vi "CR-导丝缺损检测1.vi"(8 "error in (no error)":errorcluster caption="错误输入（无错误）", 11 "名称或相对路径":string="Template Program") -> (0 "error in (no error) 2":errorcluster caption="错误输入（无错误）")   [LabVIEW 2017]
uses:
  Picture/SaveButtom.ctl
  Global System.vi
  <vilib>/Utility/xml.llb/Write to XML File(string).vi
panel:
  in  "获取图像":bool
  in  "ROI获取":bool
  in  "创建模板":bool
  in  "保存图像":bool
  out "添加的路径":path
  in  "刷新":bool
  in  "测试按钮":bool
  in  "保存按钮":bool
  in  "Main":enum32{"主参数", "模板匹配参数 ", "测试效果"}(tab)
  in  "导丝缺损检测1基础参数":T1={"IsNorImage"=TRUE, "Exposure Values"=100289, "ImagePath"=path "C:/Users/hedongpo/Desktop/514-hdp/Alignment Assemble System/Test Picture/B/3.bmp"} caption="参数界面" {"Exposure Values" scale=0.0..200000.0}
  in  "导丝缺损检测1参数":T3={"Rectangle"={"Left"=0, "Top"=0, "Right"=0, "Bottom"=0, "Rotation"=0.0}, "Algorithm "=2, "Parameters"={"Number of Matches Requested"=1, "Minimum Match Score"=800.0, "Angle Ranges"=[{"Start Angle"=-180.0, "End Angle"=180.0}]}, "Advanced Options "=[{"Item"=102, "Value"=10.0}, {"Item"=106, "Value"=300.0}, {"Item"=107, "Value"=0.0}, {"Item"=108, "Value"=6.0}, {"Item"=109, "Value"=1.0}, {"Item"=114, "Value"=25.0}, {"Item"=111, "Value"=20.0}, {"Item"=112, "Value"=10.0}, {"Item"=113, "Value"=20.0}, {"Item"=103, "Value"=1.0}, {"Item"=104, "Value"=20.0}, {"Item"=105, "Value"=0.0}, {"Item"=100, "Value"=5.0}], "模板路径"=path "", "Color Plane "=0} {"Color Plane" items=["Red", "Green", "Blue", "Hue", "Saturation", "Luminance", "Value", "Intensity"]; "Advanced Options"."Item" items=["LD Sampling - Minimum Constrast"=0, "LD Sampling - Enable Subpixel Accuracy"=1, "LD Sampling - Search Strategy"=2, "LD Sampling - Subpixel Iterations"=3, "LD Sampling - Subpixel Tolerance"=4, "LD Sampling - Initial Match List Length"=5, "LD Sampling - Match List Reduction Factor"=6, "LD Sampling - Initial Step Size"=7, "LD Sampling - Intermediate Angular Accuracy"=8, "-"=9, "Pyramid - Max Pyramid Level"=100, "Pyramid - Minimum Contrast"=102, "Pyramid - Enable Subpixel Accuracy"=103, "Pyramid - Subpixel Iterations"=104, "Pyramid - Subpixel Tolerance"=105, "Pyramid - Initial Match List Length"=106, "Pyramid - Match List Reduction Factor"=107, "Pyramid - Intermediate Angular Accuracy"=108, "Pyramid - Process Border Matches"=109, "Pyramid - Min Match Separation Distance"=111, "Pyramid - Min Match Separation Angle"=112, "Pyramid - Max Match Overlap"=113, "Pyramid - Max Cache in MB"=114, "Pyramid - Clear Cache"=115, "-"=116, "Enable Defect Map"=200]; "Algorithm" items=["All", "Low Discrepancy Sampling", "Grayscale Value Pyramid", "Gradients Pyramid"]; "Rectangle"."Rotation" format="%.2f"; "Rectangle"."Left" scale=0.0..1024.0; "Rectangle"."Right" scale=0.0..1024.0}
  out "结果":bool
  out "原始图像":T4(plugin-control)
  out "路径输出":path
  in  "Vision Paramter Save Buttom":T5
  out "system time":string
  in  "取消按钮":bool
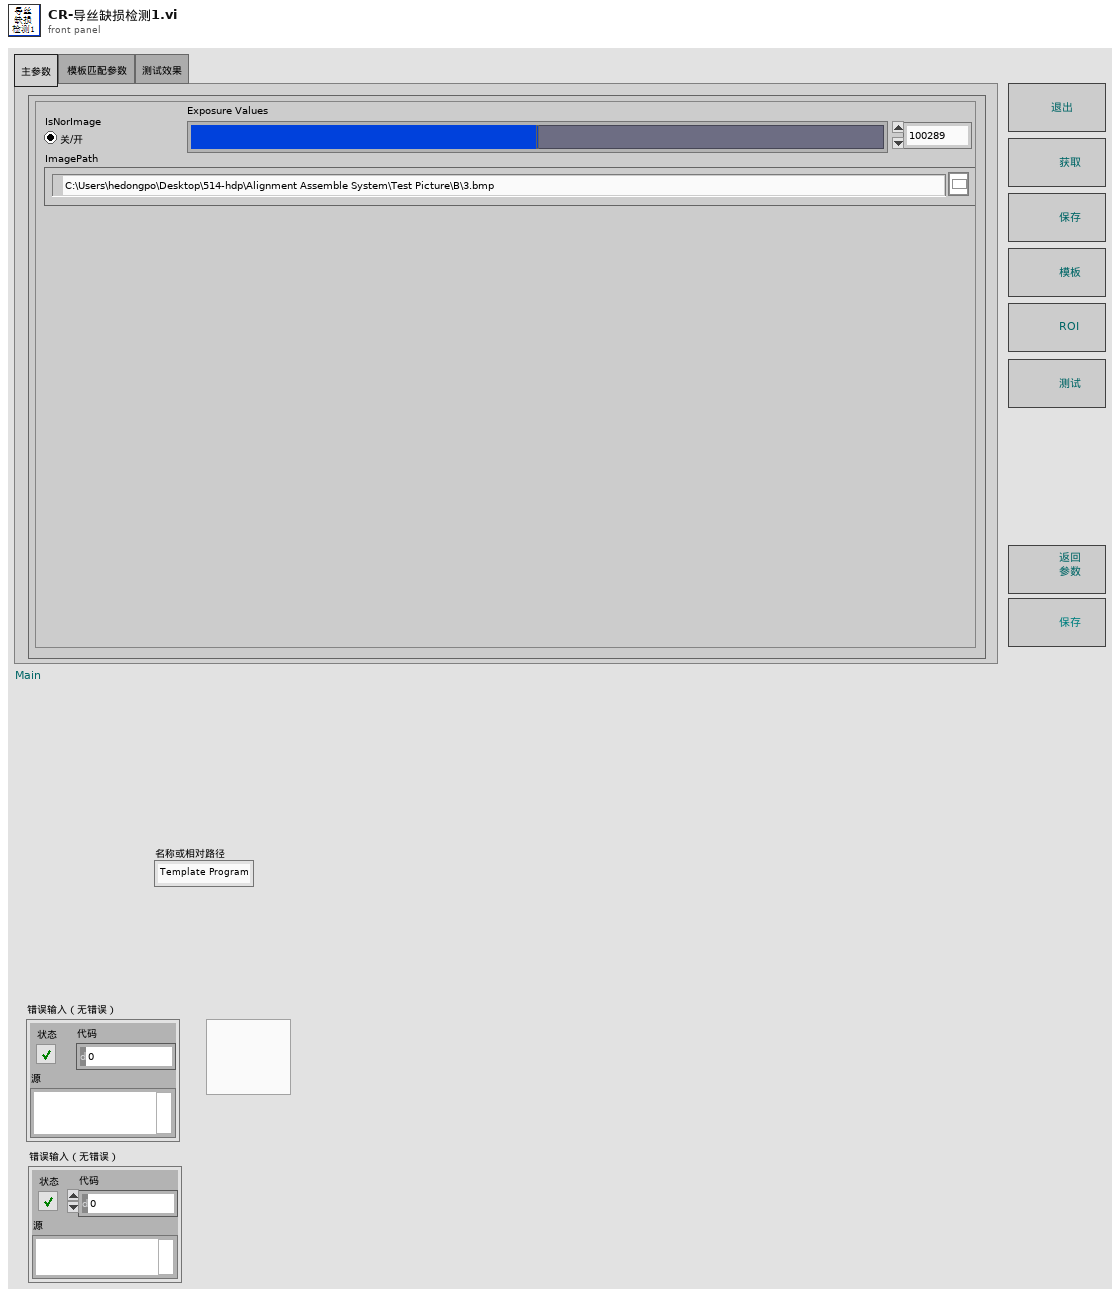
[diagram p1: front panel]
types:
  T1 = cluster{"IsNorImage":bool, "Exposure Values":u32, "ImagePath":path}
  T2 = typedef "IMAQ Rectangle" = cluster{"Left":i32, "Top":i32, "Right":i32, "Bottom":i32, "Rotation":dbl}
  T3 = cluster{"Rectangle":T2, "Algorithm ":i32, "Parameters":cluster{"Number of Matches Requested":i32, "Minimum Match Score":sgl, "Angle Ranges":cluster{"Start Angle":sgl, "End Angle":sgl}[]}, "Advanced Options ":cluster{"Item":u16, "Value":dbl}[], "模板路径":path, "Color Plane ":i32}
  T4 = typedef "IMAQ Image.ctl" = refnum<image>
  T5 = typedef "SaveButtom.ctl" = bool
  T6 = cluster{"index":i32, "this vi":refnum<vi>, "error out":errorcluster}
  T7 = cluster{"master data":string, "priority":u16, "secondary data":string[]}
  T8 = cluster{"case name":string[], "queue array":refnum<queue>[]}
  T9 = cluster{"Global Rectangle":i32[], "Contours":cluster{"Contour Type":u32, "ROI Type":u32, "Points":i32[]}[]}
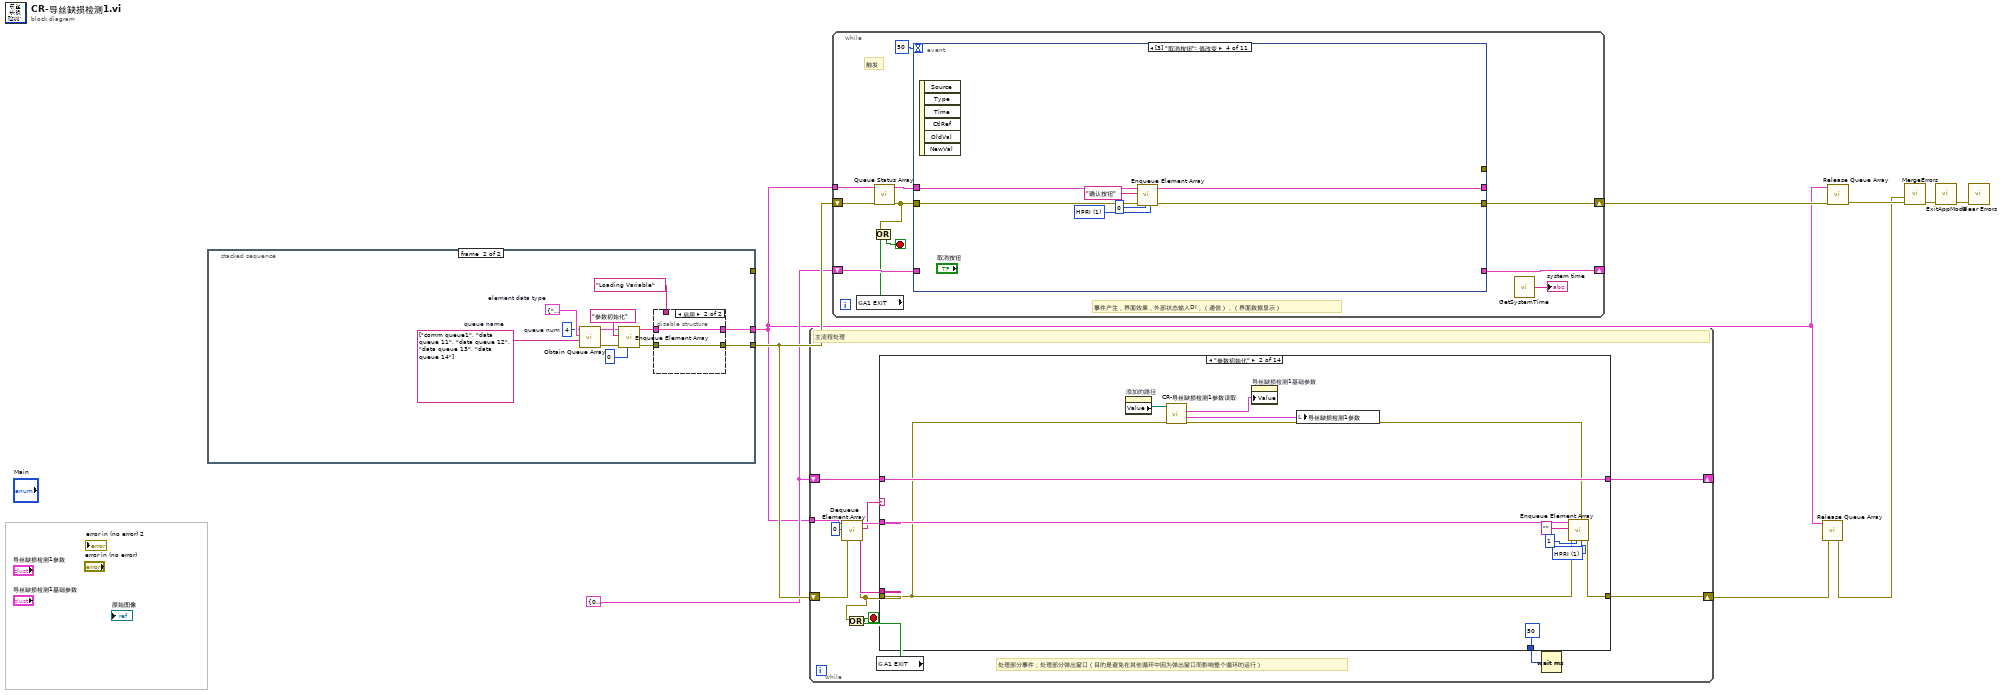
[diagram p0: block diagram]
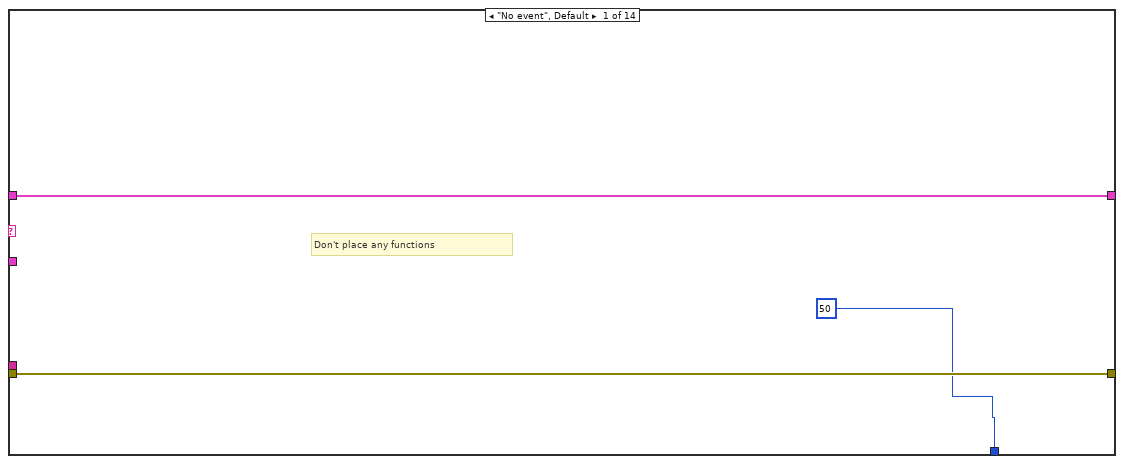
[diagram p2: hidden frame]
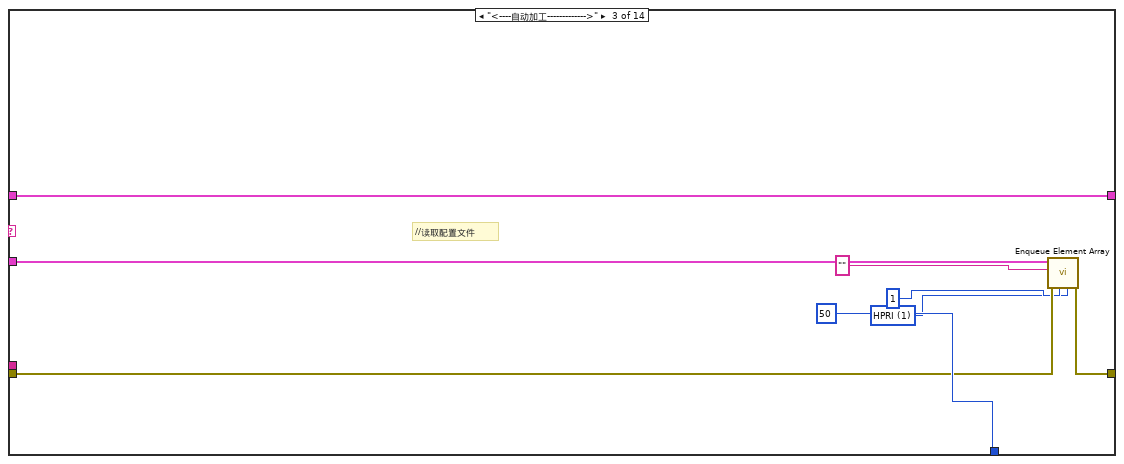
[diagram p3: hidden frame]
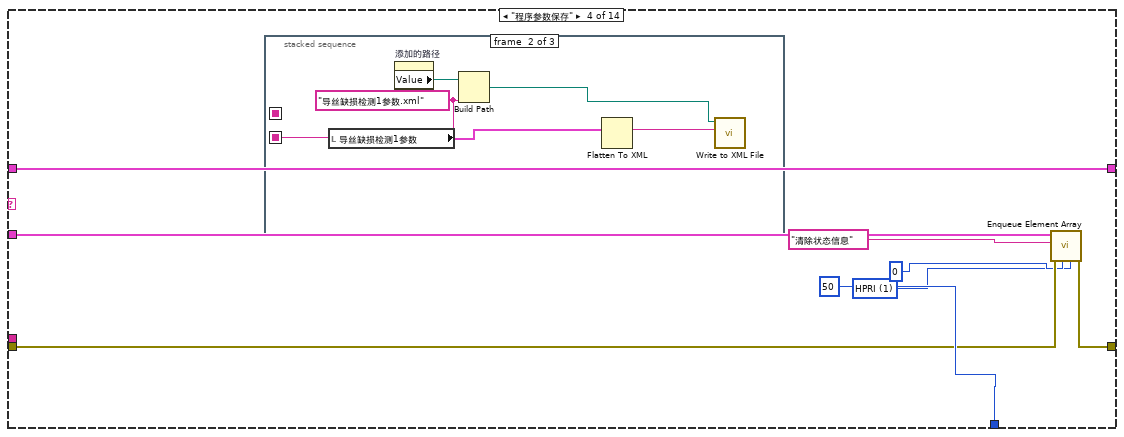
[diagram p4: hidden frame]
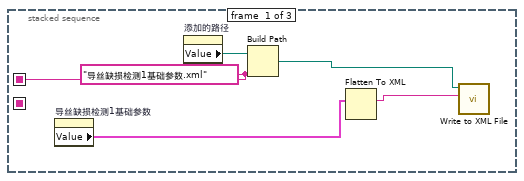
[diagram p5: hidden frame]
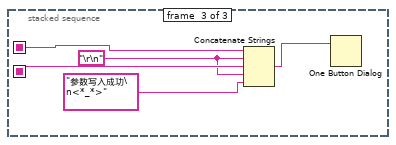
[diagram p6: hidden frame]
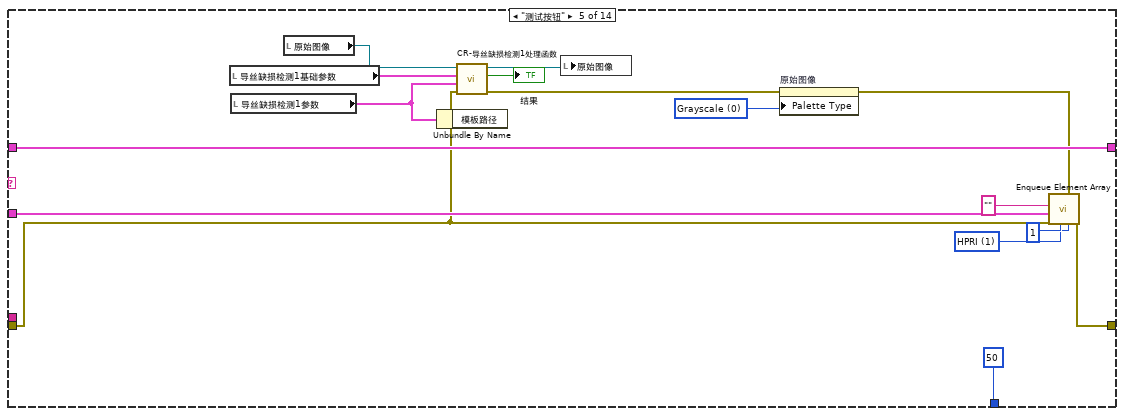
[diagram p7: hidden frame]
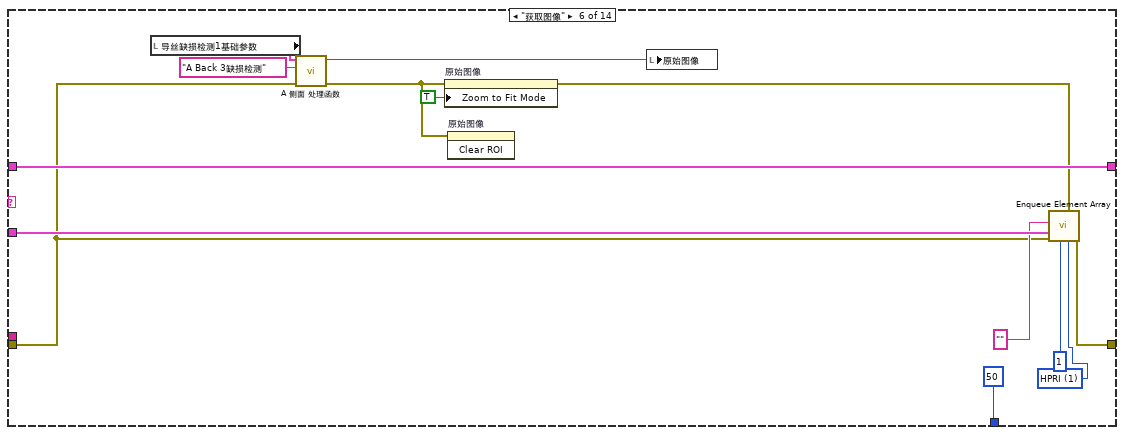
[diagram p8: hidden frame]
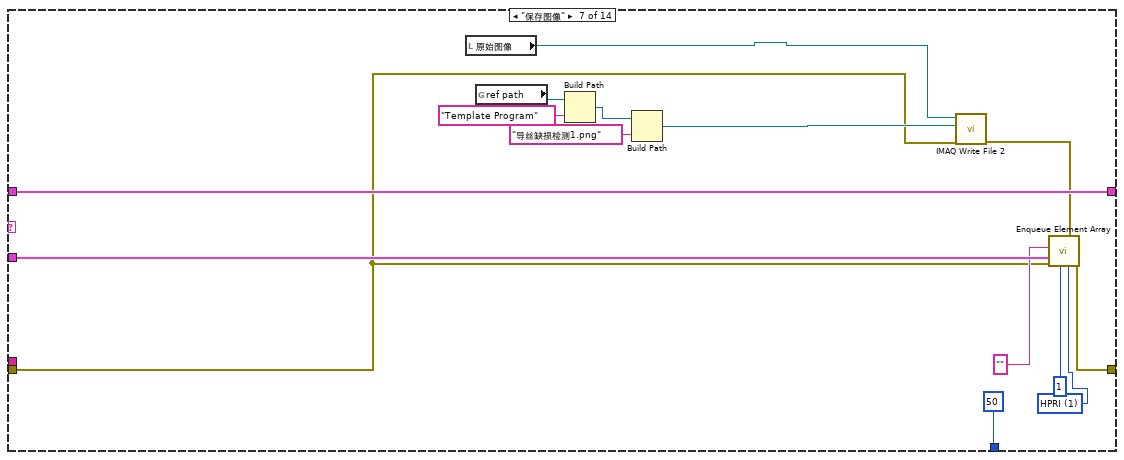
[diagram p9: hidden frame]
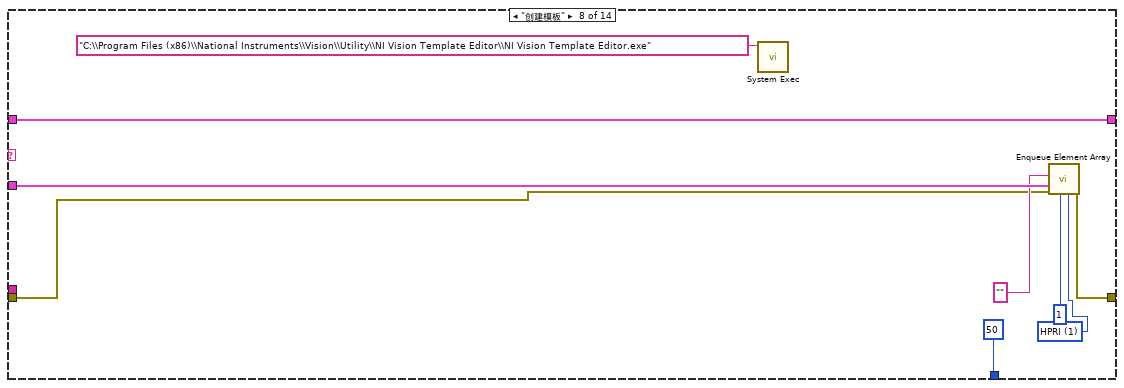
[diagram p10: hidden frame]
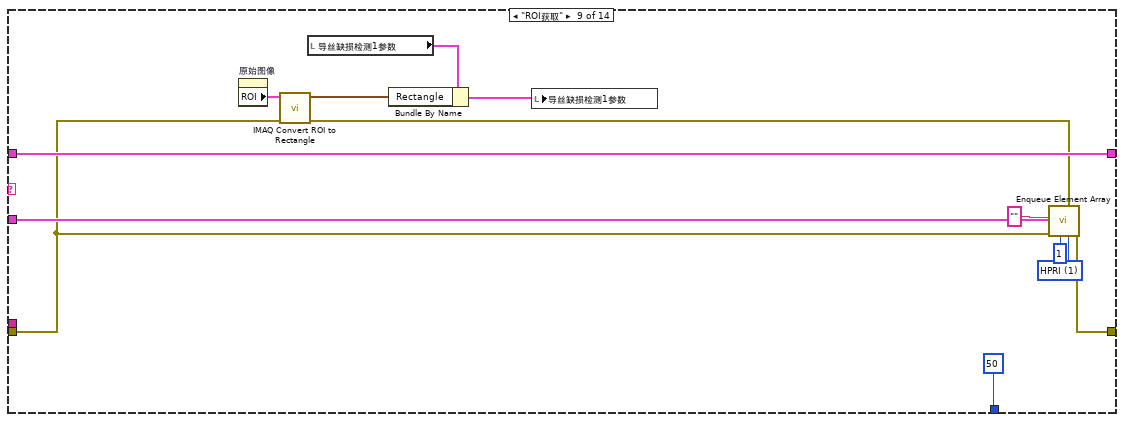
[diagram p11: hidden frame]
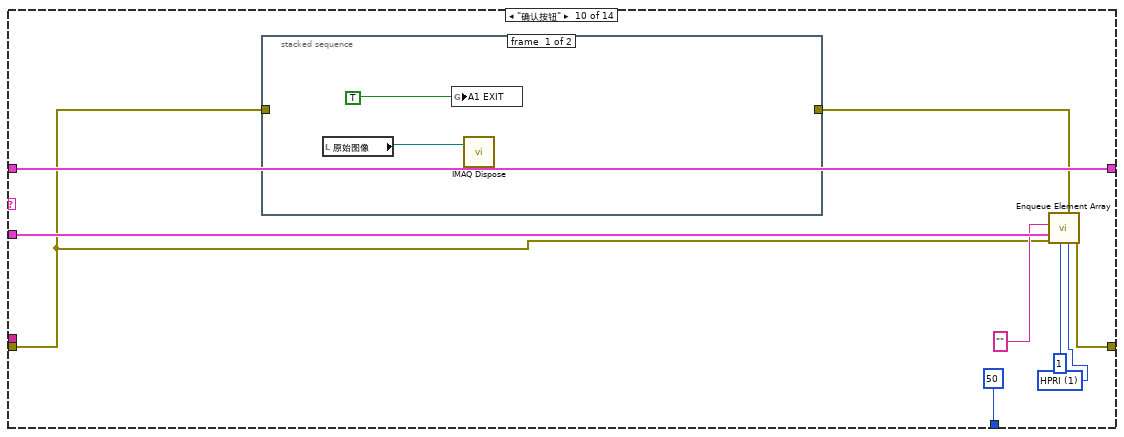
[diagram p12: hidden frame]
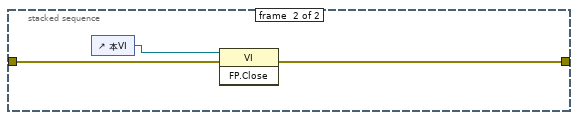
[diagram p13: hidden frame]
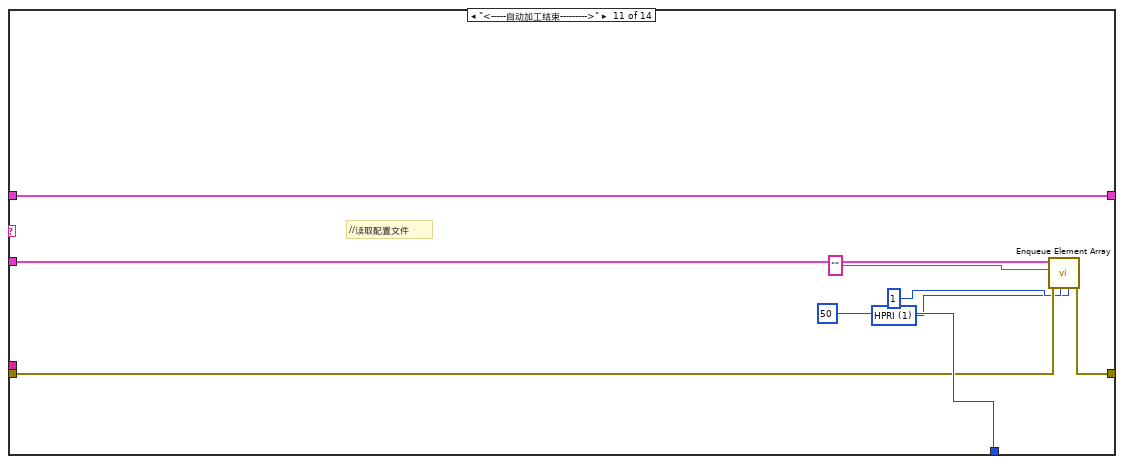
[diagram p14: hidden frame]
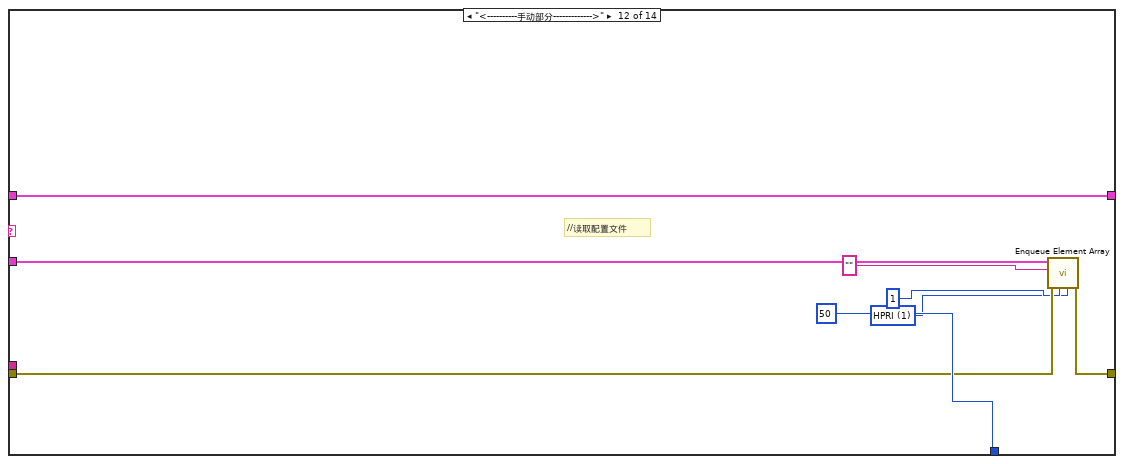
[diagram p15: hidden frame]
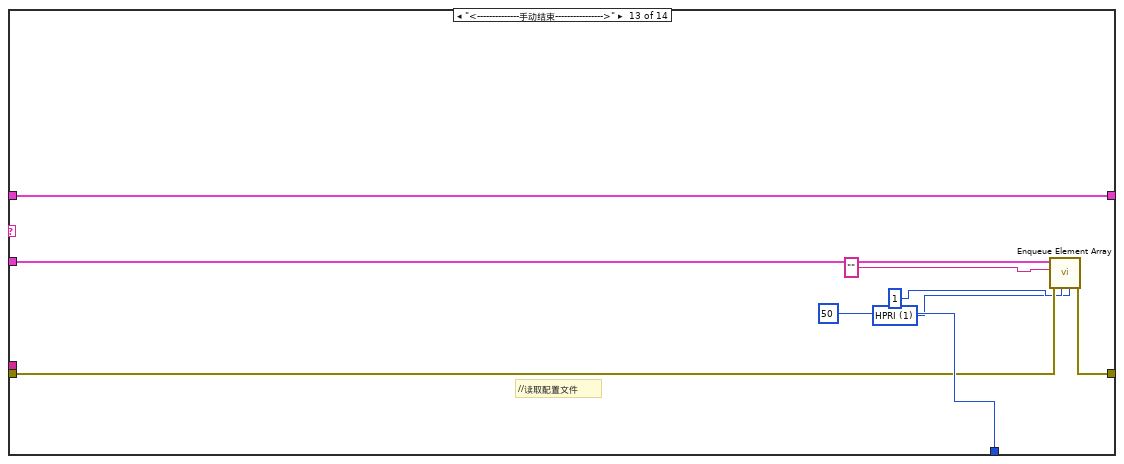
[diagram p16: hidden frame]
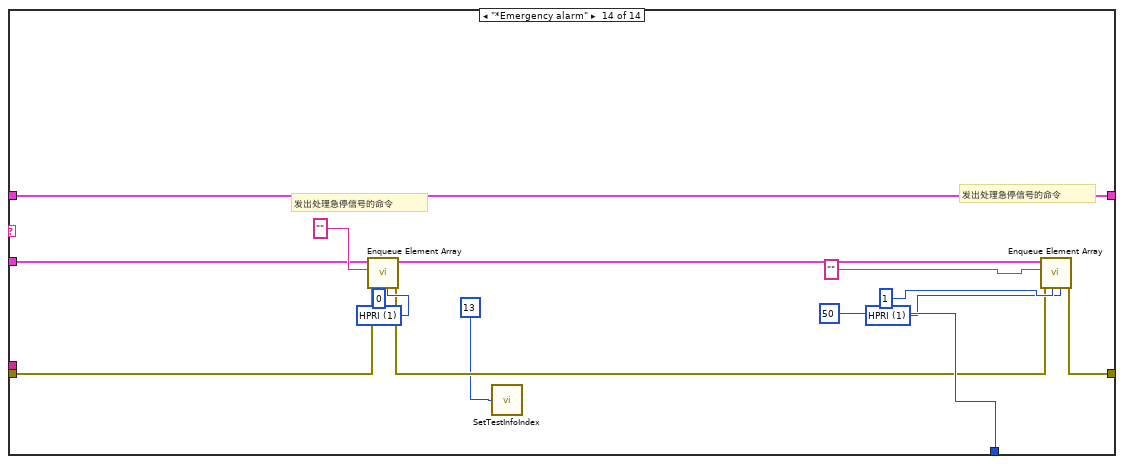
[diagram p17: hidden frame]
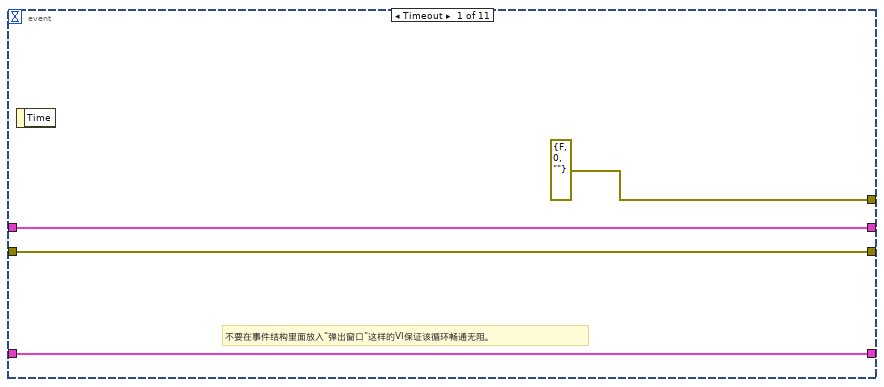
[diagram p18: hidden frame]
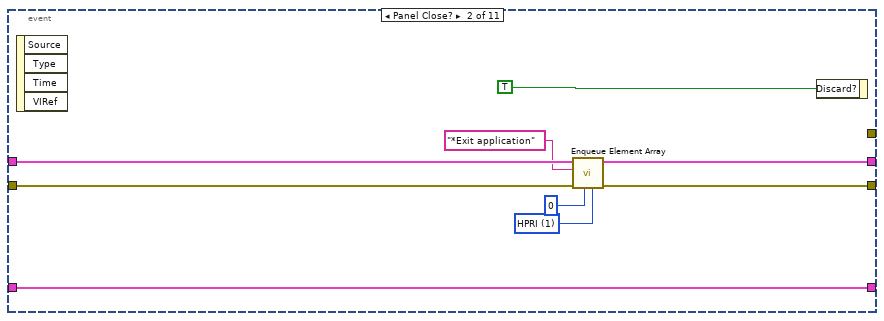
[diagram p19: hidden frame]
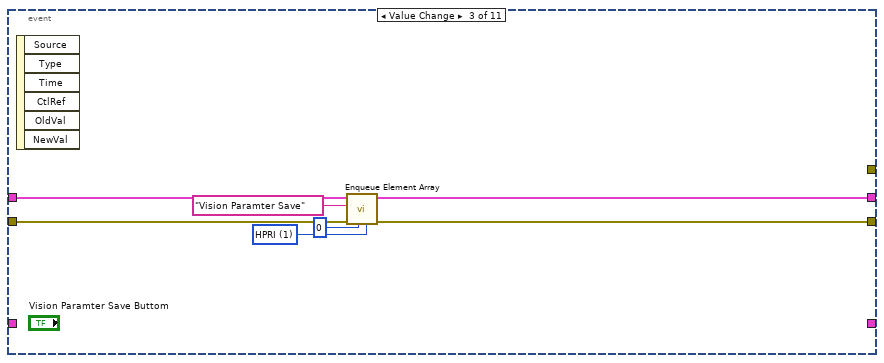
[diagram p20: hidden frame]
diagram:
  w4 = T6 {"index"=0, "this vi"=refnum, "error out"={"status"=FALSE, "code"=0, "source"=""}} ("parameter buffer")
  n1 = stacked-sequence {
    tunnel: [w15 _] -> _
    tunnel: [_ w19] -> w5
    tunnel: [_ w18] -> w1
    frame #0 {
      n2 = global read "Global System.vi" "ref path"() -> (w13:path)
      n3 = Build Path(base path=w13, name or relative path="Template Program" ("名称或相对路径")) -> (appended path=w11:path)
      n4 = property on="Main" class="TabCtl (严格)"("Value"=enum32{"主参数", "模板匹配参数 ", "测试效果"}."主参数" ("Main")) -> ()  [unwired: 2 in, 2 out]
      n5 = Build Path(base path=w11, name or relative path="名称或相对路径") -> (appended path=w17:path)
      "添加的路径" <- w17
      n6 = List Folder(path=w17) -> (path out=→"路径输出":path, error out=w15:errorcluster)  [unwired: 3 in, 2 out]
    }
    frame #1 {
      w27 = string[] ["comm queue1", "data queue 11", "data queue 12", "data queue 13", "data queue 14"]  # queue name
      w28 = 4  # queue num
      w29 = T7 {"master data"="", "priority"=0, "secondary data"=[]}  # element data type
      n7 = call "Obtain Queue Array.vi"("queue name"=w27, "element data type"=w29, "queue num"=w28) -> ("error out"=w23:errorcluster, "queue out"=w24:T8)  [unwired: 2 in, 1 out]
      n8 = call "Enqueue Element Array.vi"("queue index"=0, "error in"=w23, "master data"="参数初始化", "queue in"=w24) -> ("error out"=w22:errorcluster, "queue out"=w21:T8)  [unwired: 6 in]
      n9 = disable-structure shown="启用" {
        disable-tunnel: w22 -> [w35 w36]
        disable-tunnel: w21 -> [w34 w37]
        disable-tunnel: "Loading Variable" ("master data") -> [w33 _]
        disable-tunnel: [w31 w36] -> w19
        disable-tunnel: [w30 w37] -> w18
        frame Disabled {
          n10 = call "Enqueue Element Array.vi"("queue index"=12, "error in"=w35, "master data"=w33, "queue in"=w34) -> ("error out"=w31:errorcluster, "queue out"=w30:T8)  [unwired: 6 in]
        }
        frame Enabled {
        }
      }
    }
  }
  n11 = while {
    shift-right: [w50] -> w3
    shift-left: w5 -> [w41]
    shift-right: [w47] -> _
    shift-left: w4 -> [w48]
    tunnel: w1 -> [w43]
    stop <- w38 stop-if-true
    # "处理部分事件；处理部分弹出窗口（目的是避免在其他循环中因为弹出窗口而影响整个循环的运行）"
    # "主流程处理"
    n12 = call "Dequeue Element Array.vi"("queue in"=w43, "queue index"=0, "error in"=w41) -> ("queue out"=w46:T8, "master data"=w45:string, "secondary data"=w44:string[], "error out"=w40:errorcluster)  [unwired: 2 in, 1 out]
    n13 = global read "Global System.vi" "A1 EXIT"() -> (w39:bool)
    n14 = Or(x=w40, y=w39) -> (x .or. y?=w38:bool)
    n15 = case shown="\"参数初始化\"" w45 {
      tunnel: w46 -> [_ w64 w72 w74 w111 w125 w140 w149 w162 w171 w184 w192 w200 w206]
      tunnel: w40 -> [w52 w57 w68 w78 w104 w116 w127 w143 w155 w165 w180 w188 w196 w203]
      tunnel: [w52 w63 w71 w80 w110 w124 w139 w148 w161 w170 w183 w191 w199 w214] -> w50
      tunnel: [50 50 50 50 50 50 50 50 50 50 50 50 50 50] -> w49
      tunnel: w48 -> [w53 w59 w69 w75 w106 w120 w135 w144 w157 w166 w181 w189 w197 w212]
      tunnel: [w53 w59 w69 w75 w106 w120 w135 w144 w157 w166 w181 w189 w197 w212] -> w47
      tunnel: w44 -> [_ _ _ _ _ _ _ _ _ _ _ _ _ _]
      frame "No event", Default {
        # "Don't place any functions"
      }
      frame "参数初始化" {
        w60 = u16 1 items=["HPRI"=1, "LPRI"=0] ("priority")
        n16 = property on="添加的路径" class="Path"() -> ("Value"=w58:path)  [unwired: 2 in, 2 out]
        n17 = call "CR-导丝缺损检测1参数读取.vi"("error in (no error)"=w57, "基路径"=w58) -> ("error out"=w54:errorcluster, "导丝缺损检测1参数"=w55:T3, "导丝缺损检测1基础参数"=w56:T1)  [unwired: 6 in]
        n18 = property on="导丝缺损检测1基础参数" class="Clust (严格)"("Value"=w56) -> ()  [unwired: 2 in, 2 out]
        n19 = local write "导丝缺损检测1参数"(w55) -> ()
        n20 = call "Enqueue Element Array.vi"("priority"=w60, "device error in"=w54, "queue index"=1, "error in"=w57, "master data"="" ("Element 1"), "queue in"=w64) -> ("error out"=w63:errorcluster)  [unwired: 4 in, 1 out]
      }
      frame "<----自动加工------------->" {
        w66 = u16 1 items=["HPRI"=1, "LPRI"=0] ("priority")
        # "//读取配置文件"
        n21 = call "Enqueue Element Array.vi"("priority"=w66, "queue index"=1, "error in"=w68, "master data"="" ("Element 1"), "queue in"=w72) -> ("error out"=w71:errorcluster)  [unwired: 5 in, 1 out]
      }
      frame "程序参数保存" {
        w76 = u16 1 items=["HPRI"=1, "LPRI"=0] ("priority")
        n22 = stacked-sequence {
          seq-local: [w82 _ _] -> [_ _ w95]
          seq-local: [_ w88 _] -> [_ _ w93]
          frame #0 {
            w82 = "导丝缺损检测1基础参数.xml" ("名称或相对路径")
            n23 = property on="导丝缺损检测1基础参数" class="Clust (严格)"() -> ("Value"=w85:T1)  [unwired: 2 in, 2 out]
            n24 = property on="添加的路径" class="Path"() -> ("Value"=w86:path)  [unwired: 2 in, 2 out]
            n25 = Build Path(base path=w86, name or relative path=w82) -> (appended path=w83:path)
            n26 = Flatten To XML(anything=w85) -> (xml string=w84:string)
            n27 = call-poly <vilib>:"Write to XML File.vi"("XML Input"=w84, "XML File Path"=w83) -> ()  [unwired: 7 in, 3 out]
          }
          frame #1 {
            w88 = "导丝缺损检测1参数.xml" ("名称或相对路径")
            n28 = local read "导丝缺损检测1参数"() -> (w87:T3)
            n29 = property on="添加的路径" class="Path"() -> ("Value"=w91:path)  [unwired: 2 in, 2 out]
            n30 = Build Path(base path=w91, name or relative path=w88) -> (appended path=w89:path)
            n31 = Flatten To XML(anything=w87) -> (xml string=w90:string)
            n32 = call-poly <vilib>:"Write to XML File.vi"("XML Input"=w90, "XML File Path"=w89) -> ()  [unwired: 7 in, 3 out]
          }
          frame #2 {
            w92 = "\r\n"
            n33 = Concatenate Strings(w95, w92, w93, w92, "参数写入成功\n<*_*>" ("消息")) -> (w94:string)
            n34 = One Button Dialog(message=w94) -> ()  [unwired: 1 in, 1 out]
          }
        }
        n35 = call "Enqueue Element Array.vi"("priority"=w76, "queue index"=0, "error in"=w78, "master data"="清除状态信息" ("Element 1"), "queue in"=w74) -> ("error out"=w80:errorcluster)  [unwired: 5 in, 1 out]
      }
      frame "测试按钮" {
        w99 = u32 0 items=["Grayscale", "Binary", "Gradient", "Rainbow", "Temperature", "User Defined", "Binary 16 Bit", "Gradient 16 Bit", "Rainbow 16 Bit", "Temperature 16 Bit", "User Defined 16 Bit"] ("Palette:Palette Type")
        w107 = u16 1 items=["HPRI"=1, "LPRI"=0] ("priority")
        n36 = local read "导丝缺损检测1基础参数"() -> (w105:T1)
        n37 = local read "导丝缺损检测1参数"() -> (w102:T3)
        n38 = local read "原始图像"() -> (w101:T4)
        n39 = Unbundle By Name(w102) -> ()  [unwired: 1 out]
        n40 = call "CR-导丝缺损检测1处理函数.vi"("error in (no error)"=w104, "参数"=w102, "基础参数"=w105, "Image in"=w101) -> ("error out"=w100:errorcluster, "j结果"=→"结果":bool, "Image out"=w103:T4)  [unwired: 4 in, 1 out]
        n41 = local write "原始图像"(w103) -> ()
        n42 = property on="原始图像" class="ImageControl"(error in=w100, "Palette Type"=w99) -> (error out=w97:errorcluster)  [unwired: 1 in, 1 out]
        n43 = call "Enqueue Element Array.vi"("priority"=w107, "device error in"=w97, "queue index"=1, "error in"=w104, "master data"="" ("Element 1"), "queue in"=w111) -> ("error out"=w110:errorcluster)  [unwired: 4 in, 1 out]
      }
      frame "获取图像" {
        w121 = u16 1 items=["HPRI"=1, "LPRI"=0] ("priority")
        n44 = local read "导丝缺损检测1基础参数"() -> (w118:T1)
        n45 = call "A 侧面 处理函数.vi"("error in (no error)"=w116, "Image Name"="A Back 3缺损检测", "ParamsUI"=w118) -> ("error out"=w113:errorcluster, "Image out"=w117:T4)  [unwired: 5 in, 2 out]
        n46 = property on="原始图像" class="ImageControl"(error in=w113, "Zoom to Fit Mode"=TRUE) -> (error out=w114:errorcluster)  [unwired: 1 in, 1 out]
        n47 = invoke on="原始图像" class="ImageControl" method="Clear ROI"(error in=w113) -> ()  [unwired: 2 in, 3 out]
        n48 = local write "原始图像"(w117) -> ()
        n49 = call "Enqueue Element Array.vi"("priority"=w121, "device error in"=w114, "queue index"=1, "error in"=w116, "master data"="" ("Element 1"), "queue in"=w125) -> ("error out"=w124:errorcluster)  [unwired: 4 in, 1 out]
      }
      frame "保存图像" {
        w136 = u16 1 items=["HPRI"=1, "LPRI"=0] ("priority")
        n50 = local read "原始图像"() -> (w128:T4)
        n51 = global read "Global System.vi" "ref path"() -> (w134:path)
        n52 = Build Path(base path=w134, name or relative path="Template Program" ("名称或相对路径")) -> (appended path=w132:path)
        n53 = Build Path(base path=w132, name or relative path="导丝缺损检测1.png" ("名称或相对路径")) -> (appended path=w130:path)
        n54 = call-poly "IMAQ Write File 2"("error in (no error)"=w127, "File Path"=w130, "Image"=w128) -> ("error out"=w129:errorcluster)  [unwired: 7 in, 1 out]
        n55 = call "Enqueue Element Array.vi"("priority"=w136, "device error in"=w129, "queue index"=1, "error in"=w127, "master data"="" ("Element 1"), "queue in"=w140) -> ("error out"=w139:errorcluster)  [unwired: 4 in, 1 out]
      }
      frame "创建模板" {
        w145 = u16 1 items=["HPRI"=1, "LPRI"=0] ("priority")
        n56 = call <vilib>:"System Exec.vi"("command line"="C:\\Program Files (x86)\\National Instruments\\Vision\\Utility\\NI Vision Template Editor\\NI Vision Template Editor.exe") -> ()  [unwired: 7 in, 4 out]
        n57 = call "Enqueue Element Array.vi"("priority"=w145, "queue index"=1, "error in"=w143, "master data"="" ("Element 1"), "queue in"=w149) -> ("error out"=w148:errorcluster)  [unwired: 5 in, 1 out]
      }
      frame "ROI获取" {
        w158 = u16 1 items=["HPRI"=1, "LPRI"=0] ("priority")
        n58 = property on="原始图像" class="ImageControl"() -> ("ROI"=w156:T9)  [unwired: 2 in, 2 out]
        n59 = call "IMAQ Convert ROI to Rectangle"("error in (no error)"=w155, "ROI Descriptor"=w156) -> ("error out"=w151:errorcluster, "Rectangle"=w153:T2)  [unwired: 7 in]
        n60 = local read "导丝缺损检测1参数"() -> (w154:T3)
        n61 = Bundle By Name(cluster=w154, "Rectangle"=w153) -> (w152:T3)
        n62 = local write "导丝缺损检测1参数"(w152) -> ()
        n63 = call "Enqueue Element Array.vi"("priority"=w158, "device error in"=w151, "queue index"=1, "error in"=w155, "master data"="" ("Element 1"), "queue in"=w162) -> ("error out"=w161:errorcluster)  [unwired: 4 in, 1 out]
      }
      frame "确认按钮" {
        w167 = u16 1 items=["HPRI"=1, "LPRI"=0] ("priority")
        n64 = stacked-sequence {
          tunnel: w165 -> [_ w176]
          tunnel: [_ w175] -> w164
          frame #0 {
            n65 = local read "原始图像"() -> (w173:T4)
            n66 = global write "Global System.vi" "A1 EXIT"(TRUE ("EXIT")) -> ()
            n67 = call "IMAQ Dispose"("Image"=w173) -> ()  [unwired: 5 in, 1 out]
          }
          frame #1 {
            n68 = control-ref of="本VI"() -> (w177:refnum<vi>)
            n69 = invoke class="VI" method="FP.Close"(reference=w177, error in=w176) -> (error out=w175:errorcluster)  [unwired: 1 in, 2 out]
          }
        }
        n70 = call "Enqueue Element Array.vi"("priority"=w167, "device error in"=w164, "queue index"=1, "error in"=w165, "master data"="" ("Element 1"), "queue in"=w171) -> ("error out"=w170:errorcluster)  [unwired: 4 in, 1 out]
      }
      frame "<-----自动加工结束--------->" {
        w178 = u16 1 items=["HPRI"=1, "LPRI"=0] ("priority")
        # "//读取配置文件"
        n71 = call "Enqueue Element Array.vi"("priority"=w178, "queue index"=1, "error in"=w180, "master data"="" ("Element 1"), "queue in"=w184) -> ("error out"=w183:errorcluster)  [unwired: 5 in, 1 out]
      }
      frame "<----------手动部分------------->" {
        w186 = u16 1 items=["HPRI"=1, "LPRI"=0] ("priority")
        # "//读取配置文件"
        n72 = call "Enqueue Element Array.vi"("priority"=w186, "queue index"=1, "error in"=w188, "master data"="" ("Element 1"), "queue in"=w192) -> ("error out"=w191:errorcluster)  [unwired: 5 in, 1 out]
      }
      frame "<--------------手动结束---------------->" {
        w194 = u16 1 items=["HPRI"=1, "LPRI"=0] ("priority")
        # "//读取配置文件"
        n73 = call "Enqueue Element Array.vi"("priority"=w194, "queue index"=1, "error in"=w196, "master data"="" ("Element 1"), "queue in"=w200) -> ("error out"=w199:errorcluster)  [unwired: 5 in, 1 out]
      }
      frame "*Emergency alarm" {
        w209 = u16 1 items=["HPRI"=1, "LPRI"=0] ("priority")
        w210 = u16 1 items=["HPRI"=1, "LPRI"=0] ("priority")
        # "发出处理急停信号的命令"
        # "发出处理急停信号的命令"
        n74 = call "Enqueue Element Array.vi"("priority"=w209, "queue index"=0, "error in"=w203, "master data"="" ("Element 1"), "queue in"=w206) -> ("error out"=w204:errorcluster, "queue out"=w205:T8)  [unwired: 5 in]
        n75 = call "SetTestInfoIndex.vi"("test info index"=13) -> ()
        n76 = call "Enqueue Element Array.vi"("priority"=w210, "queue index"=1, "error in"=w204, "master data"="" ("Element 1"), "queue in"=w205) -> ("error out"=w214:errorcluster)  [unwired: 5 in, 1 out]
      }
    }
    n77 = Wait (ms)(milliseconds to wait=w49) -> ()  [unwired: 1 out]
  }
  n78 = while {
    shift-right: [w219] -> w6
    shift-left: w5 -> [w223]
    shift-right: [w221] -> _
    shift-left: w4 -> [w222]
    tunnel: w1 -> [w225]
    stop <- w216 stop-if-true
    # "触发"
    # "事件产生，界面效果，外部状态输入DI，（通信），（界面数据显示）"
    n79 = global read "Global System.vi" "A1 EXIT"() -> (w217:bool)
    n80 = call "Queue Status Array.vi"("error in (no error)"=w223, "queue in"=w225) -> ("error out"=w218:errorcluster, "queue out"=w220:T8)  [unwired: 4 in]
    n81 = Or(x=w218, y=w217) -> (x .or. y?=w216:bool)
    n82 = event shown="[3] \"取消按钮\": 值改变" {
      selector: _ -> [_ _ _ _ _ _ _ _ _ _ _]
      dyn-events: _ -> [_ _ _ _ _ _ _ _ _ _ _]
      timeout: 50 -> [_ _ _ _ _ _ _ _ _ _ _]
      tunnel: w222 -> [w230 w238 _ _ _ _ _ _ _ _ _]
      tunnel: [w230 w238 _ _ _ _ _ _ _ _ _] -> w221
      tunnel: [errorcluster {"status"=FALSE, "code"=0, "source"=""} ("error out") _ _ _ _ _ _ _ _ _ _] -> _
      tunnel: w220 -> [w228 w237 w243 w250 w257 w265 w272 w279 w287 w295 w303]
      tunnel: w218 -> [w227 w236 w242 w249 w256 w264 w271 w278 w286 w294 w302]
      tunnel: [w227 w235 w240 w247 w254 w262 w269 w276 w284 w292 w300] -> w219
      tunnel: [w228 w234 w241 w248 w255 w263 w270 w277 w285 w293 w301] -> _
      event Timeout {
        # "不要在事件结构里面放入\"弹出窗口\"这样的VI保证该循环畅通无阻。"
        n83 = event-data() -> ()  [unwired: 1 in, 1 out]
      }
      event Panel Close? {
        w232 = u16 1 items=["HPRI"=1, "LPRI"=0] ("priority")
        n84 = event-data() -> ()  [unwired: 1 in, 4 out]
        n85 = call "Enqueue Element Array.vi"("priority"=w232, "queue index"=0, "error in"=w236, "master data"="*Exit application", "queue in"=w237) -> ("error out"=w235:errorcluster, "queue out"=w234:T8)  [unwired: 5 in]
        n86 = event-data("Discard?"=TRUE) -> ()  [unwired: 1 in, 1 out]
      }
      event Value Change {
        w245 = u16 1 items=["HPRI"=1, "LPRI"=0] ("priority")
        n87 = event-data() -> ()  [unwired: 1 in, 6 out]
        n88 = call "Enqueue Element Array.vi"("priority"=w245, "queue index"=0, "error in"=w242, "master data"="Vision Paramter Save", "queue in"=w243) -> ("error out"=w240:errorcluster, "queue out"=w241:T8)  [unwired: 5 in]
      }
      event "取消按钮": Value Change {
        w252 = u16 1 items=["HPRI"=1, "LPRI"=0] ("priority")
        n89 = event-data() -> ()  [unwired: 1 in, 6 out]
        n90 = call "Enqueue Element Array.vi"("priority"=w252, "queue index"=0, "error in"=w249, "master data"="确认按钮", "queue in"=w250) -> ("error out"=w247:errorcluster, "queue out"=w248:T8)  [unwired: 5 in]
      }
      event "保存按钮": Value Change {
        w259 = u16 1 items=["HPRI"=1, "LPRI"=0] ("priority")
        n91 = event-data() -> ()  [unwired: 1 in, 6 out]
        n92 = call "Enqueue Element Array.vi"("priority"=w259, "queue index"=0, "error in"=w256, "master data"="程序参数保存", "queue in"=w257) -> ("error out"=w254:errorcluster, "queue out"=w255:T8)  [unwired: 5 in]
      }
      event "获取图像": Value Change {
        w267 = u16 1 items=["HPRI"=1, "LPRI"=0] ("priority")
        n93 = event-data() -> ()  [unwired: 1 in, 6 out]
        n94 = property on="Main" class="TabCtl (严格)"("Value"=enum32{"主参数", "模板匹配参数 ", "测试效果"}."测试效果" ("Main")) -> ()  [unwired: 2 in, 2 out]
        n95 = call "Enqueue Element Array.vi"("priority"=w267, "queue index"=0, "error in"=w264, "master data"="获取图像", "queue in"=w265) -> ("error out"=w262:errorcluster, "queue out"=w263:T8)  [unwired: 5 in]
      }
      event "保存图像": Value Change {
        w274 = u16 1 items=["HPRI"=1, "LPRI"=0] ("priority")
        n96 = event-data() -> ()  [unwired: 1 in, 6 out]
        n97 = call "Enqueue Element Array.vi"("priority"=w274, "queue index"=0, "error in"=w271, "master data"="保存图像", "queue in"=w272) -> ("error out"=w269:errorcluster, "queue out"=w270:T8)  [unwired: 5 in]
      }
      event "创建模板": Value Change {
        w281 = u16 1 items=["HPRI"=1, "LPRI"=0] ("priority")
        n98 = event-data() -> ()  [unwired: 1 in, 6 out]
        n99 = call "Enqueue Element Array.vi"("priority"=w281, "queue index"=0, "error in"=w278, "master data"="创建模板", "queue in"=w279) -> ("error out"=w276:errorcluster, "queue out"=w277:T8)  [unwired: 5 in]
      }
      event "ROI获取": Value Change {
        w289 = u16 1 items=["HPRI"=1, "LPRI"=0] ("priority")
        n100 = event-data() -> ()  [unwired: 1 in, 6 out]
        n101 = property on="Main" class="TabCtl (严格)"("Value"=enum32{"主参数", "模板匹配参数 ", "测试效果"}."模板匹配参数 " ("Main")) -> ()  [unwired: 2 in, 2 out]
        n102 = call "Enqueue Element Array.vi"("priority"=w289, "queue index"=0, "error in"=w286, "master data"="ROI获取", "queue in"=w287) -> ("error out"=w284:errorcluster, "queue out"=w285:T8)  [unwired: 5 in]
      }
      event "测试按钮": Value Change {
        w297 = u16 1 items=["HPRI"=1, "LPRI"=0] ("priority")
        n103 = event-data() -> ()  [unwired: 1 in, 6 out]
        n104 = property on="Main" class="TabCtl (严格)"("Value"=enum32{"主参数", "模板匹配参数 ", "测试效果"}."测试效果" ("Main")) -> ()  [unwired: 2 in, 2 out]
        n105 = call "Enqueue Element Array.vi"("priority"=w297, "queue index"=0, "error in"=w294, "master data"="测试按钮", "queue in"=w295) -> ("error out"=w292:errorcluster, "queue out"=w293:T8)  [unwired: 5 in]
      }
      event "刷新": Value Change {
        n106 = event-data() -> ()  [unwired: 1 in, 6 out]
        n107 = disable-structure shown="禁用" {
          disable-tunnel: w303 -> [w307 _]
          disable-tunnel: w302 -> [w306 _]
          disable-tunnel: [w305 _] -> w301
          disable-tunnel: [w304 _] -> w300
          frame Disabled {
            w309 = u16 1 items=["HPRI"=1, "LPRI"=0] ("priority")
            # "刷新"
            n108 = call "Enqueue Element Array.vi"("priority"=w309, "queue index"=0, "error in"=w306, "master data"="刷新", "queue in"=w307) -> ("error out"=w304:errorcluster, "queue out"=w305:T8)  [unwired: 5 in]
          }
          frame Enabled {
          }
        }
        n109 = property on="Main" class="TabCtl (严格)"("Value"=enum32{"主参数", "模板匹配参数 ", "测试效果"}."模板匹配参数 " ("Main")) -> ()  [unwired: 2 in, 2 out]
      }
    }
    n110 = call "GetSystemTime.vi"() -> ("date/time string"=→"system time":string)  [unwired: 7 in]
  }
  n111 = call "Release Queue Array.vi"("error in"=w3, "queue in"=w1) -> ("error out"=w2:errorcluster)  [unwired: 2 in, 3 out]
  n112 = call "Release Queue Array.vi"("error in"=w6, "queue in"=w1) -> ("error out"=w9:errorcluster)  [unwired: 2 in, 3 out]
  n113 = call "MergeErrors.vi"("error in 3 (no error)"=w2, "error in 4 (no error)"=w9) -> ("error out"=w8:errorcluster)  [unwired: 6 in]
  n114 = call "ExitAppMode.vi"("error in (no error)"=w8) -> ("error out"=w7:errorcluster)  [unwired: 10 in]
  n115 = call <vilib>:"Clear Errors.vi"("error in (no error)"=w7) -> ()  [unwired: 5 in, 2 out]
